vi "SubVI 1.vi"() -> ()   [LabVIEW 2015]
uses:
  ctlSeqFNs_SubVI 1.ctl
  ctlSeqFNs_SubVI 2.ctl
  GLOBAL -MAIN.vi
  Instance           1 15Saved   SubVI 1 .vi
panel:
  in  "Read Cycle Time":dbl=0.05 min=0.01 max=10.0 step=0.01 format="%.2f"
  out "def F":dbl[](array[numeric])
  in  "STOP":bool
  out "Main Event Message":string
  # "Parallel SubVI 1"
  # "Acquires data and Sends to SubVI 2"
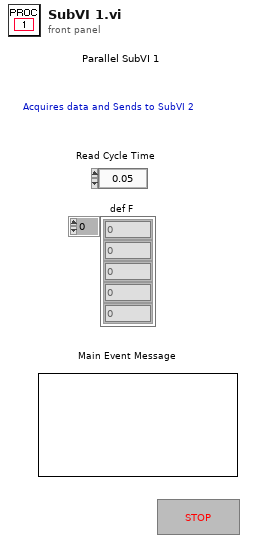
[diagram p1: front panel]
types:
  T1 = typedef "ctlSeqFNs_SubVI 1.ctl" = enum16{"INITIALIZE", "IDLE", "READ & SEND to SUBVI 2", "Main Event Msg", "ERROR", "EXIT"}
  T2 = cluster{"VIRef":refnum<vi>, "PathCurr":path, "Reads":i32, "Q2":refnum<queue>}
  T3 = typedef "ctlSeqFNs_SubVI 2.ctl" = enum16{"INITIALIZE", "IDLE", "Convert deg F to deg C", "Send to Main", "Main Event Msg", "ERROR", "EXIT"}
  T4 = enum16{"ALIGN -CENTER", "ALIGN -TOP LEFT", "ALIGN -AS IS", "ALIGN -CUSTOM"}
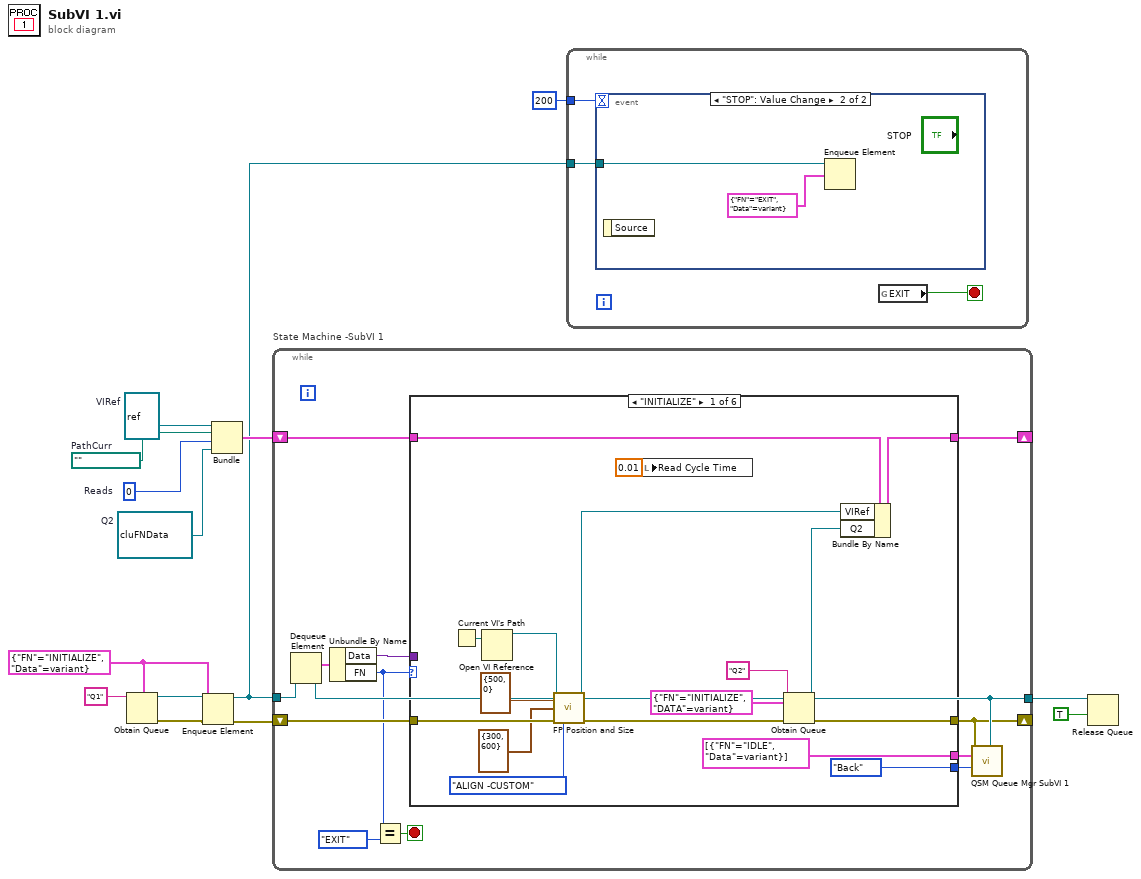
[diagram p0: block diagram]
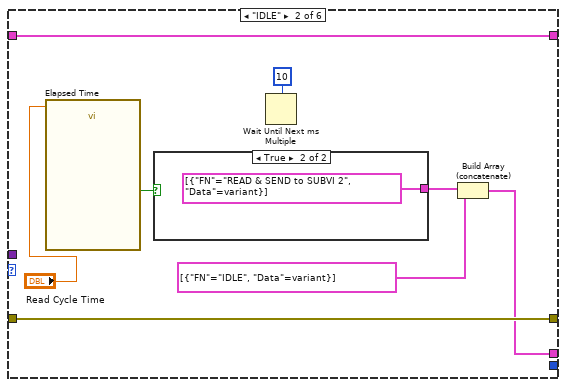
[diagram p2: hidden frame]
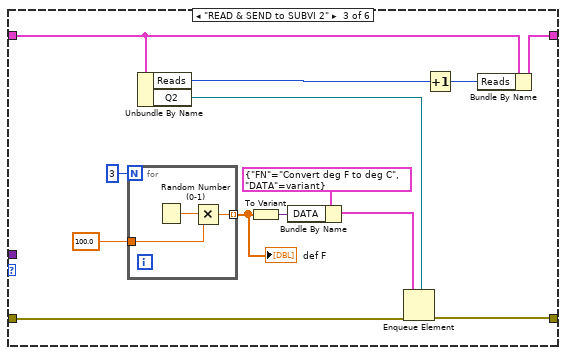
[diagram p4: hidden frame]
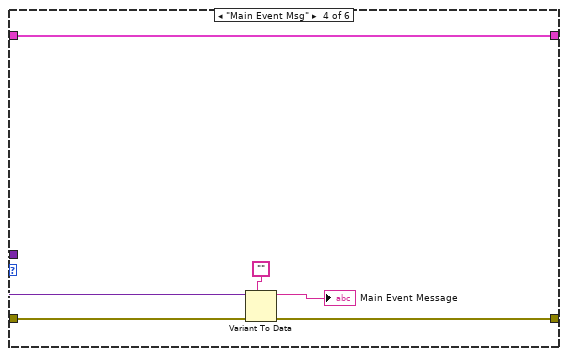
[diagram p5: hidden frame]
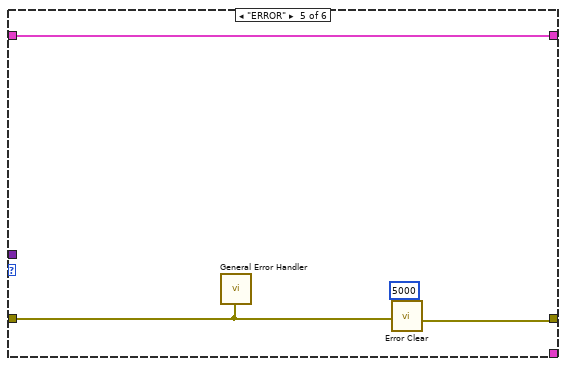
[diagram p6: hidden frame]
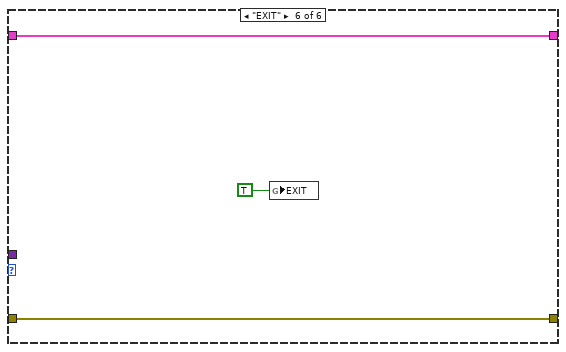
[diagram p7: hidden frame]
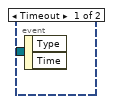
[diagram p8: hidden frame]
diagram:
  w1 = refnum<queue> refnum  # Q2
  w3 = 0  # Reads
  w7 = refnum<vi> refnum  # VIRef
  w6 = path ""  # PathCurr
  w9 = cluster{"FN":T1, "Data":variant} {"FN"=enum."INITIALIZE", "Data"=variant} ("cluFNData")
  n1 = Obtain Queue(name (unnamed)="Q1", element data type=w9) -> (queue out=w10:refnum<queue>, error out=w12:errorcluster)  [unwired: 3 in, 1 out]
  n2 = Enqueue Element(queue=w10, element=w9, error in (no error)=w12) -> (queue out=w2:refnum<queue>, error out=w11:errorcluster)  [unwired: 1 in, 1 out]
  n3 = Bundle("VIRef"=w7, "PathCurr"=w6, "Reads"=w3, "Q2"=w1) -> (w8:T2)  [unwired: 1 in]
  n4 = while "State Machine -SubVI 1" {
    shift-right: [w17] -> _
    shift-left: w11 -> [w27]
    tunnel: w2 -> [w24]
    tunnel: [w21] -> w5
    shift-right: [w18] -> _
    shift-left: w8 -> [w19]
    stop <- w26 stop-if-true
    n5 = Dequeue Element(queue=w24) -> (queue out=w21:refnum<queue>, element=w23:cluster{"FN":T1, "Data":variant})  [unwired: 2 in, 2 out]
    n6 = Unbundle By Name(w23) -> ("Data"=w22:variant, "FN"=w20:T1)
    n7 = Equal?(x=w20, y=ctlSeqFNs_SubVI_1."EXIT" ("FN")) -> (x = y?=w26:bool)
    n8 = case shown="\"INITIALIZE\"" w20 {
      tunnel: w27 -> [w39 w51 w62 w71 w76 w81]
      tunnel: [w32 w51 w61 w70 w78 w81] -> w17
      tunnel: w22 -> [_ _ _ w74 _ _]
      tunnel: w19 -> [w38 w52 w65 w75 w79 w82]
      tunnel: [w37 w52 w66 w75 w79 w82] -> w18
      tunnel: [cluster{"FN":T1, "Data":variant}[] [{"FN"=enum."IDLE", "Data"=variant}] ("QFNs") w46 _ _ _ _] -> w16
      tunnel: [enum16{"Back", "Front", "Replace"}."Back" ("Enum") _ _ _ _ _] -> w15
      frame "INITIALIZE" {
        n9 = Current VI's Path() -> (path=w42:path)
        n10 = Open VI Reference(vi path=w42) -> (vi reference=w41:refnum<vi>)  [unwired: 5 in, 1 out]
        n11 = call "FP Position and Size.vi"("VIRefNum  IN"=w41, "Poistion"=cluster{"left":i16, "top":i16} {"left"=500, "top"=0}, "Size"=cluster{"right":i16, "bottom":i16} {"right"=300, "bottom"=600}, "error in (no error)"=w39, "Mode"=T4."ALIGN -CUSTOM") -> ("VIRefNum OUT"=w40:refnum<vi>, "error out"=w33:errorcluster)  [unwired: 9 in]
        n12 = local write "Read Cycle Time"(0.01 ("Read Cycle Time")) -> ()
        n13 = Obtain Queue(name (unnamed)="Q2", element data type=cluster{"FN":T3, "DATA":variant} {"FN"=enum."INITIALIZE", "DATA"=variant} ("cluFNData"), error in (no error)=w33) -> (queue out=w29:refnum<queue>, error out=w32:errorcluster)  [unwired: 2 in, 1 out]
        n14 = Bundle By Name(cluster=w38, "VIRef"=w40, "Q2"=w29) -> (w37:T2)
      }
      frame "IDLE" {
        n15 = call "Elapsed Time"("Time Target (s)"="Read Cycle Time") -> ("Time has Elapsed"=w49:bool)  [unwired: 11 in, 7 out]
        n16 = case shown="True" w49 {
          tunnel: [_ cluster{"FN":T1, "Data":variant}[] [{"FN"=enum."READ & SEND to SUBVI 2", "Data"=variant}] ("QFNs")] -> w48
          frame False {
          }
          frame True {
          }
        }
        n17 = Wait Until Next ms Multiple(millisecond multiple=u32 10) -> ()  [unwired: 1 out]
        n18 = Build Array (concatenate)(w48, cluster{"FN":T1, "Data":variant}[] [{"FN"=enum."IDLE", "Data"=variant}] ("QFNs")) -> (w46:cluster{"FN":T1, "Data":variant}[])
      }
      frame "READ & SEND to SUBVI 2" {
        n19 = for {
          N: 3 -> [_]
          tunnel: [w68] -> w54 mode=indexing
          tunnel: 100.0 ("y") -> [w67]
          n20 = Random Number (0-1)() -> (number: 0 to 1=w69:dbl)
          n21 = Multiply(x=w69, y=w67) -> (x*y=w68:dbl)
        }
        "def F" <- w54
        n22 = Unbundle By Name(w65) -> ("Reads"=w64:i32, "Q2"=w60:refnum<queue>)
        n23 = To Variant(anything=w54) -> (Variant=w58:variant)
        n24 = Bundle By Name(cluster=cluster{"FN":T3, "DATA":variant} {"FN"=enum."Convert deg F to deg C", "DATA"=variant} ("element"), "DATA"=w58) -> (w57:cluster{"FN":T3, "DATA":variant})
        n25 = Enqueue Element(queue=w60, element=w57, error in (no error)=w62) -> (error out=w61:errorcluster)  [unwired: 1 in, 2 out]
        n26 = Increment(x=w64) -> (x+1=w63:i32)
        n27 = Bundle By Name(cluster=w65, "Reads"=w63) -> (w66:T2)
      }
      frame "Main Event Msg" {
        n28 = Variant To Data(error in=w71, type="", Variant=w74) -> (data=→"Main Event Message":string, error out=w70:errorcluster)
      }
      frame "ERROR" {
        n29 = call <vilib>:"General Error Handler.vi"("error in (no error)"=w76) -> ()  [unwired: 10 in, 5 out]
        n30 = call "Error Clear.vi"("wait(ms)"=u32 5000, "error in"=w76) -> ("error in (no error)"=w78:errorcluster)  [unwired: 6 in]
      }
      frame "EXIT" {
        n31 = global write "GLOBAL -MAIN.vi" "EXIT"(TRUE ("EXIT")) -> ()
      }
    }
    n32 = call "QSM Queue Mgr SubVI 1.vi"("QSTATES"=w16, "QRef"=w21, "Error IN"=w17, "FNs"=w15) -> ()  [unwired: 11 in, 1 out]
  }
  n33 = while "User Events SubVI 1" {
    tunnel: 200 -> [w83]
    tunnel: w2 -> [w84]
    stop <- w85 stop-if-true
    n34 = event shown="[1] \"STOP\": Value Change" {
      selector: _ -> [_ _]
      dyn-events: _ -> [_ _]
      timeout: w83 -> [_ _]
      tunnel: w84 -> [_ w87]
      event Timeout {
        n35 = event-data() -> ()  [unwired: 1 in, 2 out]
      }
      event "STOP": Value Change {
        n36 = event-data() -> ()  [unwired: 1 in, 1 out]
        n37 = Enqueue Element(queue=w87, element=cluster{"FN":T1, "Data":variant} {"FN"=enum."EXIT", "Data"=variant}) -> ()  [unwired: 2 in, 3 out]
      }
    }
    n38 = global read "GLOBAL -MAIN.vi" "EXIT"() -> (w85:bool)
  }
  n39 = Release Queue(queue=w5, force destroy? (F)=TRUE) -> ()  [unwired: 1 in, 3 out]
